vi "Get Motor Communication.vi"(8 "error in (no error)":errorcluster, 11 "wheel in":refnum<class "NI_Robotics_Wheel.lvclass">) -> (0 "error out":errorcluster, 2 "motor communication":refnum<class "NI_Robotics_Motor Communication.lvclass">, 3 "wheel out":refnum<class "NI_Robotics_Wheel.lvclass">)   [LabVIEW 2017, in "NI_Robotics_Wheel.lvclass"]
uses:
  <vilib>/robotics/Steering/Wheel/NI_Robotics_Wheel.lvclass
  <vilib>/robotics/Actuation/Motor Communication/NI_Robotics_Motor Communication.lvclass
  <vilib>/robotics/Steering/Wheel/NI_Robotics_Wheel.lvclass/NI_Robotics_Wheel.ctl
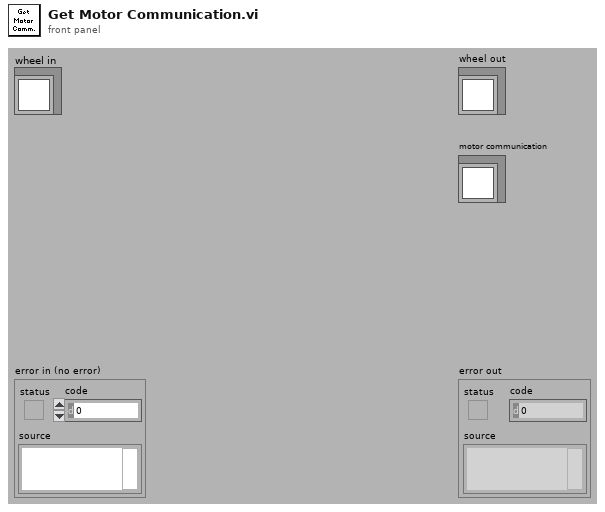
[diagram p1: front panel]
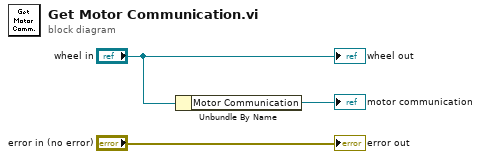
[diagram p0: block diagram]
diagram:
  n1 = Unbundle By Name("wheel in") -> ("Motor Communication"=→"motor communication":refnum<class "NI_Robotics_Motor Communication.lvclass">)
  "error out" <- "error in (no error)"
  "wheel out" <- "wheel in"
